vi "ProdaNG.CreateProcessResult.vi"(7 "Create if missing (T)":bool=TRUE, 8 "error in (no error)":errorcluster, 9 "ProcessResult":T1, 10 "ID":T2, 11 "dbHandle":i32) -> (0 "error out":errorcluster, 1 "ProcessResult 2":T1, 3 "dbHandle out":i32)   [LabVIEW 2016]
doc: "This function returns a product structure for a product, which is identified by a part and a serial number.\nImportant information: The field 'individual' was taken over from the field 'allgemein' of the legacy data directly. Because of this most products have the value 0 further on and only a few the value 1. \nParameter:\nhandle is an Integer, which is returned by the function Login() at the creation of a new connection.\nwabcoPartId is the Id of the part.\nserialNumber is the serial number of the product for the part above.\nproduct is a pointer on a product structure, which is filled if the returncode is 0. The structure must be defined in the calling program.\n\nReturncodes:\n0 No error\n< 0 ORACLE Error code\n6 (ERROR_INVALID_HANDLE) in case of an invalid handle\n1403 Record does not exist"
uses:
  Controls/ProdaNG.ProcessResult.ctl
  Controls/ProdaNG.Identification.ctl
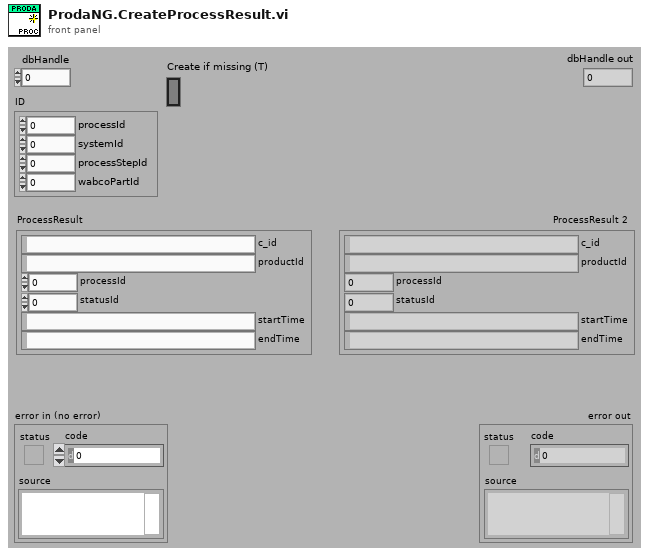
[diagram p1: front panel]
types:
  T1 = typedef "ProdaNG.ProcessResult.ctl" = cluster{"c_id":string, "productId":string, "processId":i32, "statusId":i32, "startTime":string, "endTime":string}
  T2 = typedef "ProdaNG.Identification.ctl" = cluster{"processId":i32, "systemId":i32, "processStepId":i32, "wabcoPartId":i32}
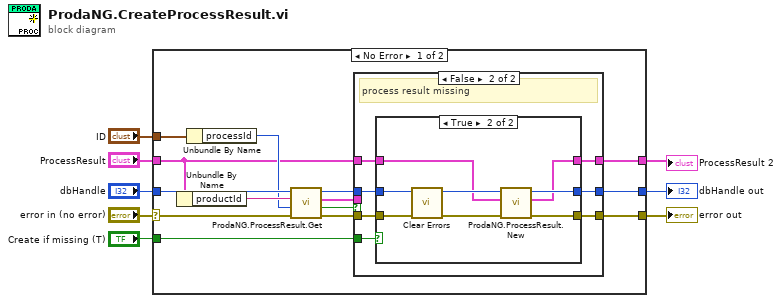
[diagram p0: block diagram]
diagram:
  n1 = case shown="No Error" "error in (no error)" {
    selector: "error in (no error)" -> [w16 w45]
    tunnel: [w14 w45] -> w7
    tunnel: "dbHandle" -> [w20 w44]
    tunnel: [w10 w44] -> w5
    tunnel: "ProcessResult" -> [w15 w43]
    tunnel: "ID" -> [w18 _]
    tunnel: [w13 w43] -> w2
    tunnel: "Create if missing (T)" -> [w9 _]
    frame No Error {
      n2 = Unbundle By Name(w15) -> ("productId"=w22:string)
      n3 = Unbundle By Name(w18) -> ("processId"=w17:i32)
      n4 = call "ProdaNG.ProcessResult.Get.vi"("error in (no error)"=w16, "processId"=w17, "productId"=w22, "dbHandle"=w20) -> ("error out"=w11:errorcluster, "Found"=w12:bool, "ProcessResult"=w19:T1, "dbHandle out"=w21:i32)  [unwired: 4 in]
      n5 = case shown="False" w12 {
        tunnel: w21 -> [w25 w32]
        tunnel: [w25 w31] -> w10
        tunnel: w19 -> [w23 _]
        tunnel: w15 -> [_ w30]
        tunnel: [w24 w28] -> w14
        tunnel: [w23 w29] -> w13
        tunnel: w11 -> [w24 w27]
        tunnel: w9 -> [_ w26]
        frame True {
          # "process result exists"
        }
        frame False {
          # "process result missing"
          n6 = case shown="True" w26 {
            tunnel: w32 -> [w34 w42]
            tunnel: [w34 w41] -> w31
            tunnel: w30 -> [w33 w39]
            tunnel: [w33 w38] -> w29
            tunnel: [w35 w37] -> w28
            tunnel: w27 -> [w35 w36]
            frame False {
            }
            frame True {
              n7 = call <vilib>:"Clear Errors.vi"("error in (no error)"=w36) -> ("error out"=w40:errorcluster)  [unwired: 5 in, 1 out]
              n8 = call "ProdaNG.ProcessResult.New.vi"("error in (no error)"=w40, "ProcessResult"=w39, "dbHandle"=w42) -> ("error out"=w37:errorcluster, "ProcessResult out"=w38:T1, "dbHandle"=w41:i32)  [unwired: 6 in]
            }
          }
        }
      }
    }
    frame Error {
    }
  }
  "error out" <- w7
  "dbHandle out" <- w5
  "ProcessResult 2" <- w2
